vi "kinetic simulation matrix-5.vi"() -> ()   [LabVIEW 2012]
uses:
  <vilib>/Utility/file.llb/Write To Spreadsheet File (DBL).vi
panel:
  in  "Fraction%":dbl=80.0 format="%#_2f"
  in  "kAF(um)2":dbl=0.24 format="%#_6f"
  in  "k2 2":dbl=0.1 format="%#_7f"
  in  "kF(um)2":dbl=0.064 format="%#_6f"
  in  "X2":dbl=0.04
  in  "one/two rates":bool
  out "Efficency Summery Full":dbl[][](graph)=[[69.9, 86.0, 91.0, 95.4, 99.0], [79.3, 86.3, 92.9, 96.5, 97.0], [88.0, 89.8, 91.4, 93.1, 95.0], [90.0, 89.7, 90.6, 91.9, 91.5], [69.9, 86.0, 91.0, 95.4, 99.0], [79.3, 86.3, 92.9, 96.5, 97.0], [88.0, 89.8, 91.4, 93.1, 95.0], [90.0, 89.7, 90.6, 91.9, 91.5]]
  in  "Transition Matrix":i32[][](array[numeric])=[[1, 1, 2, 3, 3], [5, 2, 2, 3, 4], [0, 1, 3, 3, 4], [0, 0, 5, 4, 4], [1, 1, 2, 3, 3], [0, 1, 2, 2, 5], [0, 1, 1, 3, 4], [0, 0, 5, 4, 4]]
  in  "TP - S5":dbl[][](array[numeric])=[[999.0, 0.0, 0.0], [0.0, 0.0, 0.0], [0.0, 0.0, 0.0], [0.0, 0.0, 0.0], [999.0, 0.0, 0.0], [0.0, 0.0, 111.0], [0.0, 0.0, 0.0], [0.0, 0.0, 0.0]]
  in  "TP - S4":dbl[][](array[numeric])=[[0.0, 0.0, 0.0], [0.0, 0.0, 0.0], [0.0, 0.0, 0.0], [0.0, 111.0, 0.0], [0.0, 0.0, 0.0], [111.0, 0.0, 0.0], [0.0, 0.0, 0.0], [0.0, 111.0, 0.0]]
  in  "TP - S3":dbl[][](array[numeric])=[[0.0, 0.0, 0.0], [0.0, 0.0, 0.0], [0.0, 999.0, 0.0], [0.0, 0.0, 111.0], [0.0, 0.0, 0.0], [0.0, 0.0, 0.0], [999.0, 0.0, 0.0], [0.0, 0.0, 111.0]]
  in  "TP - S2":dbl[][](array[numeric])=[[0.0, 0.0, 0.0], [0.0, 111.0, 0.0], [0.0, 0.0, 0.0], [111.0, 0.0, 0.0], [0.0, 0.0, 0.0], [0.0, 0.0, 0.0], [0.0, 0.0, 0.0], [111.0, 0.0, 0.0]]
  in  "TP - S1":dbl[][](array[numeric])=[[0.0, 999.0, 0.0], [0.0, 0.0, 111.0], [0.0, 0.0, 0.0], [0.0, 0.0, 0.0], [0.0, 999.0, 0.0], [0.0, 0.0, 0.0], [0.0, 0.0, 0.0], [0.0, 0.0, 0.0]]
  in  "Start":bool
  in  "STOP All":bool
  out "kAF'":dbl=0.048
  in  "kAF(um)":dbl=0.24 format="%#_6f"
  out "Simulated-Efficencys":dbl[][](array[numeric])=[[76.9028871391076, 99.60629921259843, 100.13123359580052, 100.13123359580052, 100.13123359580052], [96.43835616438356, 100.13698630136987, 100.13698630136987, 100.13698630136987, 100.13698630136987], [100.0, 100.11223344556679, 100.11223344556679, 100.11223344556679, 100.11223344556679], [100.08403361344537, 100.08403361344537, 100.08403361344537, 100.08403361344537, 100.08403361344537]]
  in  "State to Observe":i32=4
  in  "incubation time":dbl[](array[numeric])=[30.0, 100.0, 300.0, 1000.0, 3000.0] caption="Incubation time"
  in  "concentration (uM)":dbl[](array[numeric])=[0.2, 0.5, 1.0, 10.0]
  in  "Experamental-Efficencys":dbl[][](array[numeric])=[[69.9, 86.0, 91.0, 95.4, 99.0], [79.3, 86.3, 92.9, 96.5, 97.0], [88.0, 89.8, 91.4, 93.1, 95.0], [90.0, 89.7, 90.6, 91.9, 91.5]]
  out "Efficency Summery":dbl[][](graph)=[[69.9, 86.0, 91.0, 95.4, 99.0], [79.3, 86.3, 92.9, 96.5, 97.0], [88.0, 89.8, 91.4, 93.1, 95.0], [90.0, 89.7, 90.6, 91.9, 91.5], [28.980974719833203, 71.68360698462341, 97.88897576231432, 99.70028668230388, 99.70028668230388], [79.3, 86.3, 92.9, 96.5, 97.0], [88.0, 89.8, 91.4, 93.1, 95.0], [90.0, 89.7, 90.6, 91.9, 91.5]]
  in  "k2":dbl=0.135 format="%#_6f"
  out "AF/F":bool=TRUE
  in  "Matrix-Antifuel":dbl[][](array[numeric])=[[0.0, 0.0, 0.0, 0.0, 0.0, 0.0, 0.0, 0.0, 0.0, 0.0], [0.0, 0.0, 0.0, 0.0, 0.0, 0.0, 0.0, 0.0, 0.0, 0.0], [0.0, 0.0, 0.0, 0.0, 0.0, 0.0, 0.0, 0.0, 0.0, 0.0], [0.0, 0.0, 0.0, 0.0, 0.0, 0.0, 0.0, 0.0, 0.0, 0.0], [0.048, 0.0, 0.0, 0.0, 0.0, 0.0, 0.0, 0.0, 0.0, 0.0], [0.0, 0.0, 0.0, 0.0, 0.0, 0.0, 0.0, 0.0, 0.0, 0.0]]
  out "Concen (um)":dbl=0.2
  in  "kF(um)":dbl=0.064 format="%#_6f"
  out "kF'X":dbl=0.0005120000000000001
  in  "X":dbl=0.04
  out "kF'":dbl=0.0128
  out "nnew 2":i32=1
  out "inew 2":i32=1
  out "index_top 2":i32=2
  out "Final_A_index 2":i32[](array[numeric])=[0, 1, 2, 5, 2, 0, 0, 0, 0, 0]
  out "Final_D_index 2":i32[](array[numeric])=[0, 2, 1, 1, 4, 0, 0, 0, 0, 0]
  out "rate 2":dbl[](array[numeric])=[0.0, 0.0, 0.0, 0.0, 4000000000.000001, 0.0, 0.0, 0.0, 0.0, 0.0]
  in  "Matrix-Fuel":dbl[][](array[numeric])=[[0.0, 0.0, 0.0, 0.0, 0.0, 0.0, 0.0, 0.0, 0.0, 0.0], [0.0128, 0.0, 0.0, 0.0, 0.0, 0.0, 0.0, 0.0, 0.0, 0.0], [0.0005120000000000001, 0.0, 0.0, 0.0, 0.0, 0.0, 0.0, 0.0, 0.0, 0.0], [0.0, 0.0005120000000000001, 0.0128, 0.0, 0.0, 0.0, 0.0, 0.0, 0.0, 0.0], [0.0, 0.25, 0.25, 0.0, 0.0, 0.0, 0.0, 0.0, 0.0, 0.0], [0.0, 0.0, 0.0, 0.0, 0.0, 0.0, 0.0, 0.0, 0.0, 0.0]]
  in  "save?":bool
  out "nnew":i32=1
  out "inew":i32=1
  out "index_top":i32=2
  out "photime":dbl=9999.0
  out "srate":dbl
  out "time 2":dbl=0.30115000000000003
  out "Final_A_index":i32[](array[numeric])=[0, 1, 2, 5, 2, 0, 0, 0, 0, 0]
  out "Final_D_index":i32[](array[numeric])=[0, 2, 1, 1, 4, 0, 0, 0, 0, 0]
  out "rate":dbl[](array[numeric])=[0.0, 0.0, 0.0, 0.0, 333333000.0, 0.0, 0.0, 0.0, 0.0, 0.0]
  out "X-axes":dbl[](array[numeric])
  in  "time max":dbl=3000.0
  out "Kinetics":dbl[][](graph)
  in  "time per bin":dbl=0.1
  in  "NEXT":bool
  in  "number of state obs":i32=5
  out "Current pos":i32=5
  in  "start pos":i32
  out "probabilty distribution":dbl[](graph)=[573985.2993294162, 29260.075592117602, 1121.7302167399819, 69888.30850277809, 22353744.586358897, 0.0, 0.0, 0.0, 0.0, 0.0, 0.0, 0.0, 0.0]
  out "time":dbl=3000.0 format="%.3e"
  in  "stop inside":bool
  # "B"
  # "B"
  # "C'"
  # "D"
  # "C'"
  # "D"
  # "A"
  # "B'"
  # "A"
  # "B'"
  # "A"
  # "A"
  # "B"
  # "B"
  # "B'"
  # "B'"
  # "FUEL"
  # "C'"
  # "kF'"
  # "C'"
  # "D"
  # "ANTI-FUEL"
  # "D"
  # "kF'x"
  # "kF'"
  # "kF'x"
  # "k2"
  # "k2"
  # "200 nM"
  # "500 nM"
  # "1 uM"
  # "10 uM"
  # "30s"
  # "300s"
  # "3000s"
  # "100s"
  # "1000s"
  # "S1"
  # "S0"
  # "S2"
  # "S3"
  # "S4"
  # "999 - fuel efficency"
  # "111 antifuel efficency"
  # "F2"
  # "AF1"
  # "F3"
  # "AF2"
  # "F2"
  # "AF3"
  # "F1"
  # "AF2"
  # "right"
  # "lost"
  # "left"
  # "right"
  # "lost"
  # "left"
  # "right"
  # "lost"
  # "left"
  # "right"
  # "lost"
  # "right"
  # "lost"
  # "left"
  # "left"
  # "F2"
  # "F2"
  # "F2"
  # "F2"
  # "F2"
  # "AF1"
  # "AF1"
  # "AF1"
  # "AF1"
  # "AF1"
  # "F3"
  # "F3"
  # "F3"
  # "F3"
  # "F3"
  # "AF2"
  # "AF2"
  # "AF2"
  # "AF2"
  # "AF2"
  # "F2"
  # "F2"
  # "F2"
  # "F2"
  # "F2"
  # "AF3"
  # "AF3"
  # "AF3"
  # "AF3"
  # "AF3"
  # "F1"
  # "F1"
  # "F1"
  # "F1"
  # "F1"
  # "k1 B->D"
  # "AF2"
  # "AF2"
  # "AF2"
  # "AF2"
  # "AF2"
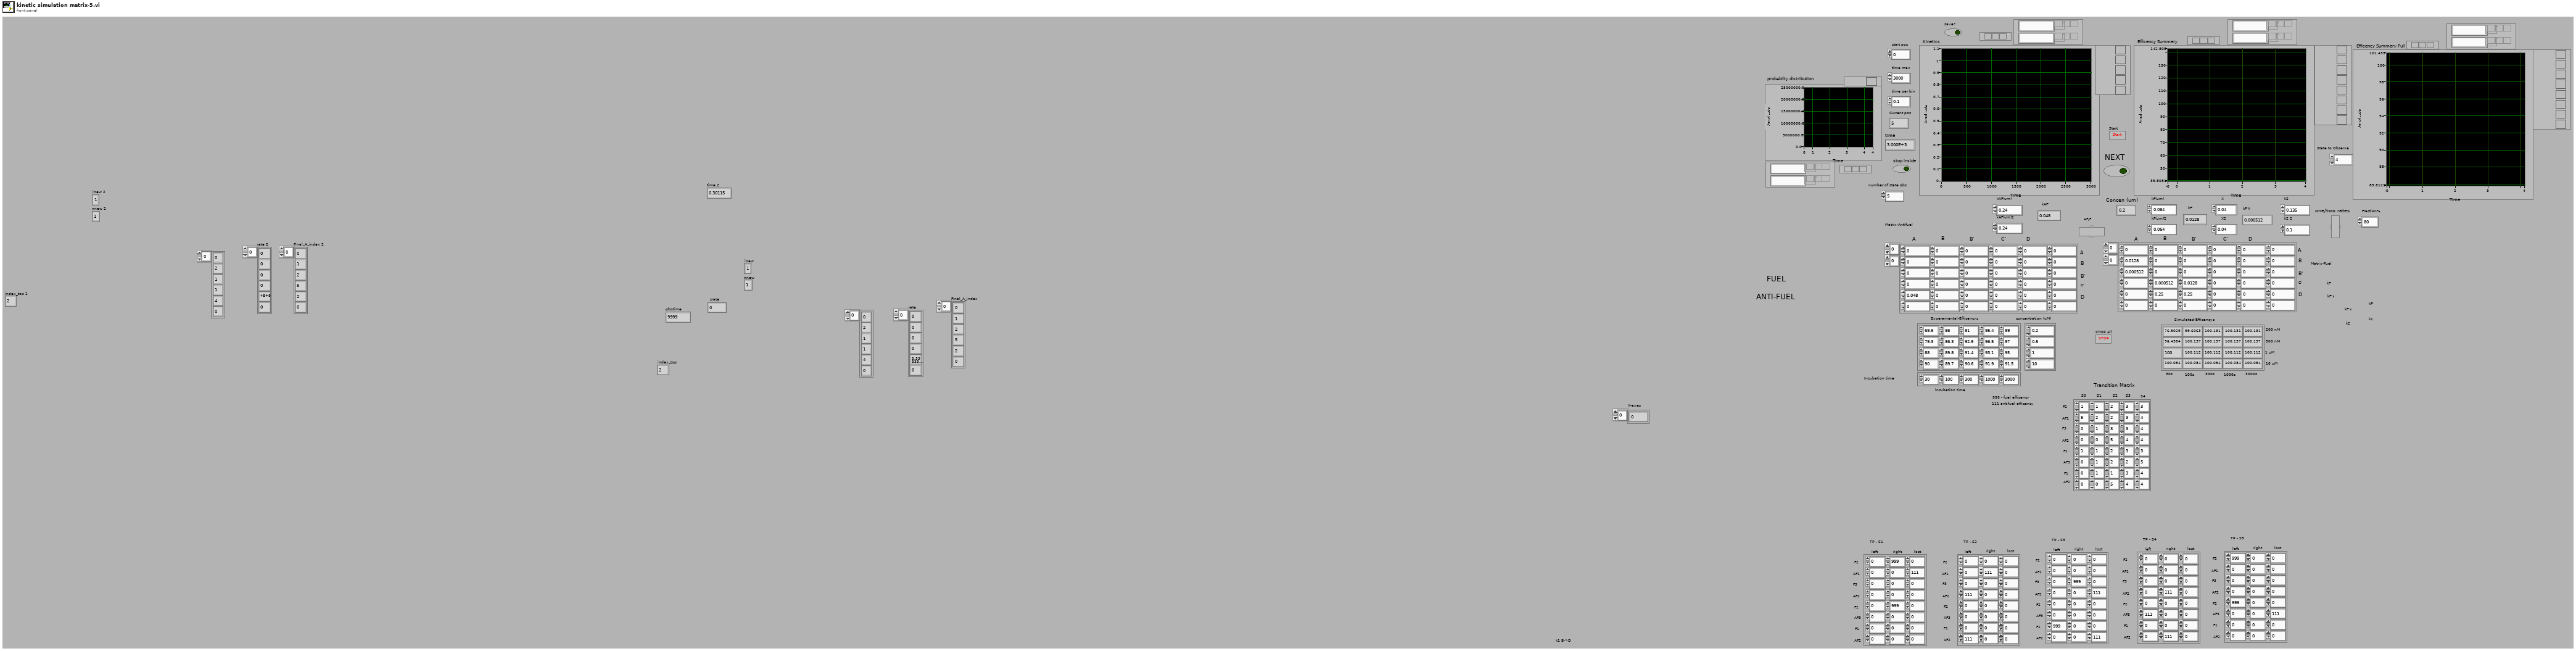
[diagram p1: front panel]
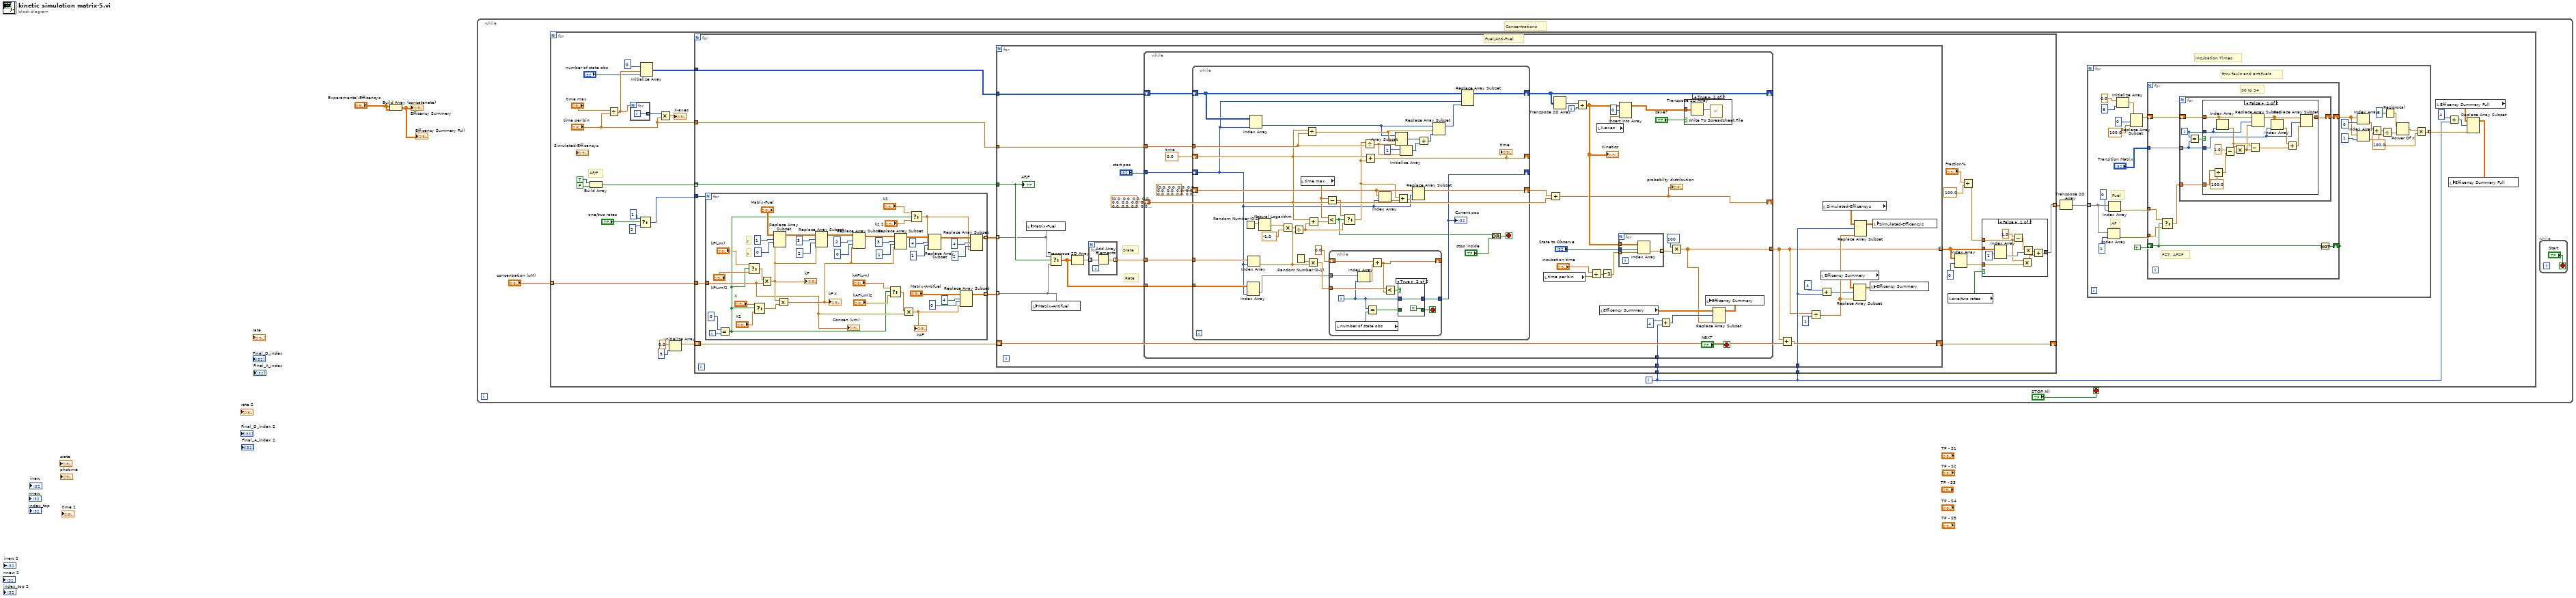
[diagram p0: block diagram]
diagram:
  n1 = Build Array (concatenate)("Experamental-Efficencys", "Experamental-Efficencys") -> (→"Efficency Summery" →"Efficency Summery Full":dbl[][])
  n2 = while {
    stop <- "STOP All" stop-if-true
    # "Concentrations"
    n3 = for {
      tunnel: "concentration (uM)" -> [w32] mode=indexing
      i -> [w10]
      # "AF/F"
      # "Incubation Times"
      n4 = Build Array(TRUE ("AF/F"), FALSE ("AF/F")) -> (w29:bool[])
      n5 = Divide(x="time max", y="time per bin") -> (x/y=w24:dbl)
      n6 = for {
        N: w24 -> [_]
        tunnel: [w276] -> w22 mode=indexing
        i -> [w276]
      }
      n7 = Select(t=1, s="one/two rates", f=2) -> (s? t:f=w11:i32)
      n8 = Initialize Array(0 ("dimension size"), w24, "number of state obs") -> (w13:i32[][])
      n9 = Multiply(x=w22, y="time per bin") -> (x*y=→"X-axes":dbl[])
      n10 = Initialize Array(0.0 ("element"), 5 ("dimension size")) -> (w20:dbl[])
      n11 = for {
        tunnel: w32 -> [w51]
        tunnel: w29 -> [w50] mode=indexing
        tunnel: w10 -> [w38]
        tunnel: [w39] -> w16 mode=indexing
        tunnel: w13 -> [w48]
        tunnel: "time per bin" -> [w47]
        shift-right: [w46] -> _
        shift-left: w20 -> [w49]
        tunnel: w11 -> [w43]
        tunnel: w10 -> [w42]
        # "Fuel/Anti-Fuel"
        n12 = for {
          N: w43 -> [_]
          tunnel: w51 -> [w73]
          tunnel: [w86] -> w45 mode=indexing
          tunnel: [w82] -> w44 mode=indexing
          i -> [w78]
          # "y"
          # "x"
          n13 = Equal?(x=0, y=w78) -> (x = y?=w63:bool)
          n14 = Select(t="kF(um)", s=w63, f="kF(um)2") -> (s? t:f=w74:dbl)
          n15 = Select(t="X", s=w63, f="X2") -> (s? t:f=w70:dbl)
          n16 = Multiply(x=w74, y=w73) -> (x*y=w80:dbl)
          "kF'" <- w80
          n17 = Replace Array Subset(array="Matrix-Fuel", new element=w80, index (row)=1, index (col)=0 ("disabled index (col)")) -> (w100:dbl[][])
          n18 = Multiply(x=w80, y=w70) -> (x*y=w81:dbl)
          "kF'X" <- w81
          n19 = Replace Array Subset(array=w100, new element=w80, index (row)=3, index (col)=2 ("disabled index (col)")) -> (w94:dbl[][])
          n20 = Replace Array Subset(array=w94, new element=w81, index (row)=2, index (col)=0 ("disabled index (col)")) -> (w95:dbl[][])
          n21 = Select(t="kAF(um)", s=w63, f="kAF(um)2") -> (s? t:f=w64:dbl)
          n22 = Replace Array Subset(array=w95, new element=w81, index (row)=3, index (col)=1 ("disabled index (col)")) -> (w88:dbl[][])
          n23 = Multiply(x=w64, y=w73) -> (x*y=w79:dbl)
          "kAF'" <- w79
          n24 = Select(t="k2", s=w63, f="k2 2") -> (s? t:f=w68:dbl)
          n25 = Replace Array Subset(array=w88, new element=w68, index (row)=4, index (col)=1 ("disabled index (col)")) -> (w89:dbl[][])
          n26 = Replace Array Subset(array="Matrix-Antifuel", new element=w79, index (row)=4, index (col)=0 ("disabled index (col)")) -> (w82:dbl[][])
          n27 = Replace Array Subset(array=w89, new element=w68, index (row)=4, index (col)=2 ("disabled index (col)")) -> (w86:dbl[][])
          "Concen (um)" <- w73
        }
        n28 = for {
          tunnel: w50 -> [w120]
          tunnel: w47 -> [w126]
          tunnel: w48 -> [w125]
          shift-right: [w112] -> w46
          shift-left: w49 -> [w119]
          tunnel: w42 -> [w107]
          tunnel: [w105] -> w41 mode=indexing
          tunnel: w45 -> [w109] mode=indexing
          tunnel: w44 -> [w108] mode=indexing
          tunnel: w38 -> [w106]
          # "Rate"
          # "Srate"
          n29 = local write "Matrix-Fuel"(w109) -> ()
          n30 = local write "Matrix-Antifuel"(w108) -> ()
          n31 = Select(t=w109, s=w120, f=w108) -> (s? t:f=w121:dbl[][])
          n32 = Transpose 2D Array(2D array=w121) -> (transposed array=w124:dbl[][])
          n33 = for {
            tunnel: w124 -> [w128] mode=indexing
            tunnel: [w129] -> w123 mode=indexing
            n34 = Add Array Elements(numeric array=w128) -> (sum=w129:dbl)
          }
          n35 = while {
            shift-right: [w131] -> _
            shift-left: dbl[] [0.0, 0.0, 0.0, 0.0, 0.0, 0.0, 0.0, 0.0, 0.0, 0.0, 0.0, 0.0, 0.0] ("Output Array") -> [w160]
            tunnel: w126 -> [w157]
            shift-right: [w154] -> _
            shift-left: w125 -> [w158]
            tunnel: w123 -> [w148]
            tunnel: w121 -> [w147]
            tunnel: "start pos" -> [w146]
            tunnel: [w132] -> w105
            tunnel: w106 -> [w130]
            i -> [w145]
            stop <- "NEXT" stop-if-true
            w156 = 0.0  # time
            n36 = while {
              shift-left: dbl[] [0.0, 0.0, 0.0, 0.0, 0.0, 0.0, 0.0, 0.0, 0.0, 0.0, 0.0, 0.0, 0.0] ("Output Array") -> [w200]
              shift-right: [w181] -> w153
              shift-left: w156 -> [w184]
              shift-right: [w179] -> _
              shift-left: w146 -> [w174]
              shift-right: [w170] -> _
              tunnel: w157 -> [w195]
              shift-right: [w182] -> w154
              shift-left: w158 -> [w188]
              tunnel: w148 -> [w176]
              tunnel: w147 -> [w175]
              stop <- w168 stop-if-true
              n37 = Random Number (0-1)() -> (number: 0 to 1=w205:dbl)
              n38 = Index Array(array=w175, index (col)=w174) -> (element=w171:dbl[])  [unwired: 1 in]
              n39 = Index Array(array=w176, index=w174) -> (element=w177:dbl)
              n40 = Index Array(array=w188, index (col)=w174) -> (element=w189:i32[])  [unwired: 1 in]
              n41 = Natural Logarithm(1:w205) -> (0:w204:dbl)
              n42 = Multiply(x=w204, y=-1.0) -> (x*y=w202:dbl)
              n43 = Divide(x=w202, y=w177) -> (x/y=w178:dbl)
              n44 = Random Number (0-1)() -> (number: 0 to 1=w201:dbl)
              n45 = local read "time max"() -> (w185:dbl)
              n46 = Divide(x=w184, y=w195) -> (x/y=w191:dbl)
              n47 = Multiply(x=w201, y=w177) -> (x*y=w172:dbl)
              n48 = Add(x=w184, y=w178) -> (x+y=w186:dbl)
              n49 = Less?(x=w185, y=w186) -> (x < y?=w169:bool)
              n50 = Subtract(x=w185, y=w184) -> (x-y=w183:dbl)
              n51 = while {
                shift-right: [w212] -> _
                shift-left: 0.0 -> [w215]
                tunnel: w172 -> [w213]
                tunnel: w171 -> [w209]
                tunnel: [w206] -> w170
                i -> [w208]
                stop <- w210 stop-if-true
                n52 = local read "number of state obs"() -> (w207:i32)
                n53 = Index Array(array=w209, index=w208) -> (element=w216:dbl)
                n54 = Equal?(x=w208, y=w207) -> (x = y?=w211:bool)
                n55 = Add(x=w215, y=w216) -> (x+y=w212:dbl)
                n56 = Less?(x=w213, y=w212) -> (x < y?=w214:bool)
                n57 = case shown="True" w214 {
                  tunnel: w208 -> [w217 w219]
                  tunnel: w211 -> [w218 _]
                  tunnel: [w218 TRUE] -> w210
                  tunnel: [w217 w219] -> w206
                  frame False {
                  }
                  frame True {
                  }
                }
              }
              "Current pos" <- w170
              n58 = Select(t=w183, s=w169, f=w178) -> (s? t:f=w180:dbl)
              n59 = Divide(x=w180, y=w195) -> (x/y=w190:dbl)
              n60 = Add(x=w184, y=w180) -> (x+y=w179:dbl)
              "time" <- w179
              n61 = Index Array(array=w200, index=w174) -> (element=w198:dbl)
              n62 = Array Subset(array=w189, index=w191, length=w190) -> (w194:i32[])
              n63 = Add(x=w180, y=w198) -> (x+y=w199:dbl)
              n64 = Initialize Array(1 ("dimension size"), w190) -> (w193:i32[])
              n65 = Replace Array Subset(array=w200, new element=w199, index=w174) -> (w181:dbl[])
              n66 = Add(x=w194, y=w193) -> (x+y=w192:i32[])
              n67 = Replace Array Subset(array=w189, new element=w192, index=w191) -> (w187:i32[])
              n68 = Replace Array Subset(array=w188, new element=w187, index (col)=w174) -> (w182:i32[][])  [unwired: 1 in]
              n69 = Or(x=w169, y="stop inside") -> (x .or. y?=w168:bool)
            }
            n70 = local read "time per bin"() -> (w141:dbl)
            n71 = Add(x=w153, y=w160) -> (x+y=w131:dbl[])
            "probabilty distribution" <- w131
            n72 = Transpose 2D Array(2D array=w154) -> (transposed array=w155:i32[][])
            n73 = Divide(x=w155, y=w145) -> (x/y=w142:dbl[][])
            "Kinetics" <- w142
            n74 = Divide(x="incubation time", y=w141) -> (x/y=w140:dbl[])
            n75 = local read "X-axes"() -> (w149:dbl[])
            n76 = local read "Efficency Summery"() -> (w144:dbl[][])
            n77 = Decrement(x=w140) -> (x-1=w138:dbl[])
            n78 = for {
              tunnel: w138 -> [w165] mode=indexing
              tunnel: [w164] -> w137 mode=indexing
              tunnel: "State to Observe" -> [w163]
              tunnel: w142 -> [w162]
              n79 = Index Array(array=w162, index (row)=w163, index (col)=w165) -> (element=w164:dbl)
            }
            n80 = Insert Into Array(array=w142, index (row)=0, new element=w149) -> (w151:dbl[][])  [unwired: 1 in]
            n81 = Add(x=4 ("index (row)"), y=w130) -> (x+y=w134:i32)
            n82 = Multiply(x=100 ("index (row)"), y=w137) -> (x*y=w132:dbl[])
            n83 = case shown="True" "save?" {
              tunnel: w151 -> [_ w167]
              frame False {
              }
              frame True {
                n84 = Transpose 2D Array(2D array=w167) -> (transposed array=w166:dbl[][])
                n85 = call-poly <vilib>:"Write To Spreadsheet File.vi"("2D data"=w166) -> ()  [unwired: 7 in, 1 out]
              }
            }
            n86 = Replace Array Subset(array=w144, new element=w132, index (row)=w134) -> (w136:dbl[][])  [unwired: 1 in]
            n87 = local write "Efficency Summery"(w136) -> ()
          }
          n88 = Add(x=w105, y=w119) -> (x+y=w112:dbl[])
          n89 = Divide(x=w105, y=1 ("index (row)")) -> (x/y=w111:dbl[])
          n90 = local read "Efficency Summery"() -> (w116:dbl[][])
          n91 = Add(x=4 ("index (row)"), y=w107) -> (x+y=w110:i32)
          n92 = local read "Simulated-Efficencys"() -> (w114:dbl[][])
          n93 = Replace Array Subset(array=w116, new element=w111, index (row)=w110) -> (w118:dbl[][])  [unwired: 1 in]
          n94 = Replace Array Subset(array=w114, new element=w111, index (row)=w107) -> (w115:dbl[][])  [unwired: 1 in]
          n95 = local write "Efficency Summery"(w118) -> ()
          n96 = local write "Simulated-Efficencys"(w115) -> ()
          "AF/F" <- w120
        }
        n97 = local read "one/two rates"() -> (w34:bool)
        n98 = Index Array(array=w41, index (row)=0 ("y")) -> (element=w33:dbl[])  [unwired: 1 in]
        n99 = Divide(x="Fraction%", y=100.0) -> (x/y=w35:dbl)
        n100 = case shown="False" w34 {
          tunnel: w41 -> [w61 _]
          tunnel: [w55 w62] -> w39
          tunnel: w35 -> [w52 _]
          tunnel: w33 -> [w53 w62]
          frame False {
            n101 = Index Array(array=w61, index (row)=1 ("y")) -> (element=w59:dbl[])  [unwired: 1 in]
            n102 = Subtract(x=1.0 ("element"), y=w52) -> (x-y=w58:dbl)
            n103 = Multiply(x=w52, y=w53) -> (x*y=w54:dbl[])
            n104 = Multiply(x=w58, y=w59) -> (x*y=w56:dbl[])
            n105 = Add(x=w56, y=w54) -> (x+y=w55:dbl[])
          }
          frame True {
          }
        }
      }
      n106 = Transpose 2D Array(2D array=w16) -> (transposed array=w9:dbl[][])
      n107 = for {
        tunnel: w9 -> [w236] mode=indexing
        tunnel: [w221] -> w15 mode=indexing
        w222 = 100.0 ("element")
        # "thru feuls and antifuels"
        # "AF"
        # "Fuel"
        n108 = Index Array(array=w236, index=1 ("disabled index (col)")) -> (element=w233:dbl)
        n109 = Index Array(array=w236, index=0 ("disabled index (col)")) -> (element=w238:dbl)
        n110 = Initialize Array(0.0 ("element"), 6 ("dimension size")) -> (w243:dbl[])
        n111 = Replace Array Subset(array=w243, new element=100.0 ("element"), index=0) -> (w240:dbl[])
        n112 = for {
          shift-right: [w247] -> w226
          shift-left: w240 -> [w248]
          tunnel: "Transition Matrix" -> [w253] mode=indexing
          tunnel: w238 -> [w251]
          tunnel: w233 -> [w250]
          shift-right: [w252] -> _
          shift-left: TRUE ("s") -> [w246]
          # "S0 to S4"
          # "F=T, AF=F"
          n113 = Select(t=w251, s=w246, f=w250) -> (s? t:f=w249:dbl)
          n114 = for {
            tunnel: w253 -> [w255] mode=indexing
            tunnel: w249 -> [w258]
            shift-right: [w254] -> w247
            shift-left: w248 -> [w257]
            i -> [w256]
            n115 = Equal?(x=w256, y=w255) -> (x = y?=w259:bool)
            n116 = case shown="False" w259 {
              tunnel: w258 -> [w274 _]
              tunnel: w257 -> [w272 w275]
              tunnel: w256 -> [w271 _]
              tunnel: w255 -> [w263 _]
              tunnel: [w261 w275] -> w254
              frame False {
                n117 = Divide(x=w274, y=100.0 ("element")) -> (x/y=w270:dbl)
                n118 = Index Array(array=w272, index=w271) -> (element=w267:dbl)
                n119 = Subtract(x=1.0, y=w270) -> (x-y=w268:dbl)
                n120 = Multiply(x=w267, y=w268) -> (x*y=w266:dbl)
                n121 = Subtract(x=w267, y=w266) -> (x-y=w260:dbl)
                n122 = Replace Array Subset(array=w272, new element=w266, index=w271) -> (w262:dbl[])
                n123 = Index Array(array=w262, index=w263) -> (element=w265:dbl)
                n124 = Add(x=w265, y=w260) -> (x+y=w264:dbl)
                n125 = Replace Array Subset(array=w262, new element=w264, index=w263) -> (w261:dbl[])
              }
              frame True {
                # "Stay at the same state"
              }
            }
          }
          n126 = Not(x=w246) -> (.not. x?=w252:bool)
        }
        n127 = Index Array(array=w226, index=0 ("index (row)")) -> (element=w228:dbl)
        n128 = Index Array(array=w226, index=1 ("index (row)")) -> (element=w227:dbl)
        n129 = Add(x=w228, y=w227) -> (x+y=w225:dbl)
        n130 = Divide(x=w225, y=w222) -> (x/y=w224:dbl)
        n131 = Reciprocal(x=8 ("index (row)")) -> (1/x=w232:dbl)
        n132 = Power Of X(1:w224, 2:w232) -> (0:w223:dbl)
        n133 = Multiply(x=w223, y=w222) -> (x*y=w221:dbl)
      }
      n134 = local read "Efficency Summery Full"() -> (w19:dbl[][])
      n135 = Add(x=4 ("index (row)"), y=w10) -> (x+y=w17:i32)
      n136 = Replace Array Subset(array=w19, new element=w15, index (row)=w17) -> (w14:dbl[][])  [unwired: 1 in]
      n137 = local write "Efficency Summery Full"(w14) -> ()
    }
    n138 = while {
      stop <- "Start" stop-if-true
    }
  }
